vi "STATUS List (SubVI).vi"(0 "ESP Config":T1={"COM Port Input"="COM8", "Manual Command"={"Device Type"="", "Instance"="", "Command"="", "Sub-Command"="", "Parameters (Seperate by :)"=""}, "Device Type"="e", "Instance"="a", "Use Manual Command"=FALSE, "Timeout [msec]"=1000, "Read/Write Wait [msec]"=50}, 5 "Command Table Ref":refnum<vi>, 7 "STATUS Display Ref":refnum<vi>, 9 "STATUS Command Ref":refnum<vi>) -> (10 "Status Data":string, 15 "STATUS List":errorcluster)   [LabVIEW 2011]
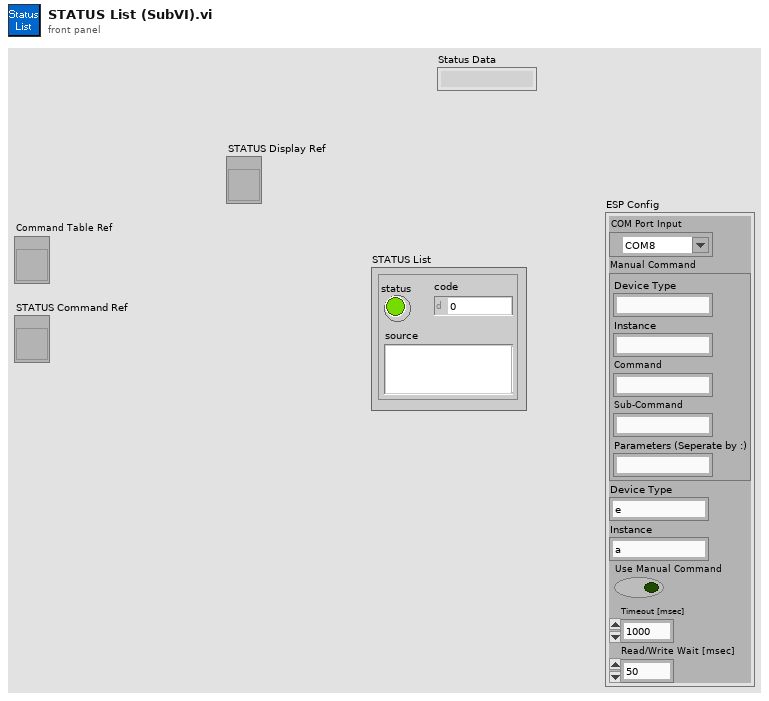
[diagram p1: front panel]
types:
  T1 = cluster{"COM Port Input":refnum<visa-resource-name>, "Manual Command":cluster{"Device Type":string, "Instance":string, "Command":string, "Sub-Command":string, "Parameters (Seperate by :)":string}, "Device Type":string, "Instance":string, "Use Manual Command":bool, "Timeout [msec]":u32, "Read/Write Wait [msec]":u32}
  T2 = cluster{"Device Type":string, "Instance":string, "Command":string, "Sub-Command":string, "Parameters (Seperate by :)":string}
  T3 = cluster{"Write Command":string, "Read String":string, "Read Bytes":u32, "Bytes at Port":u32, "Response":string, "ACK":bool, "EOT":bool, "NAK":bool, "Parameters":string[]}
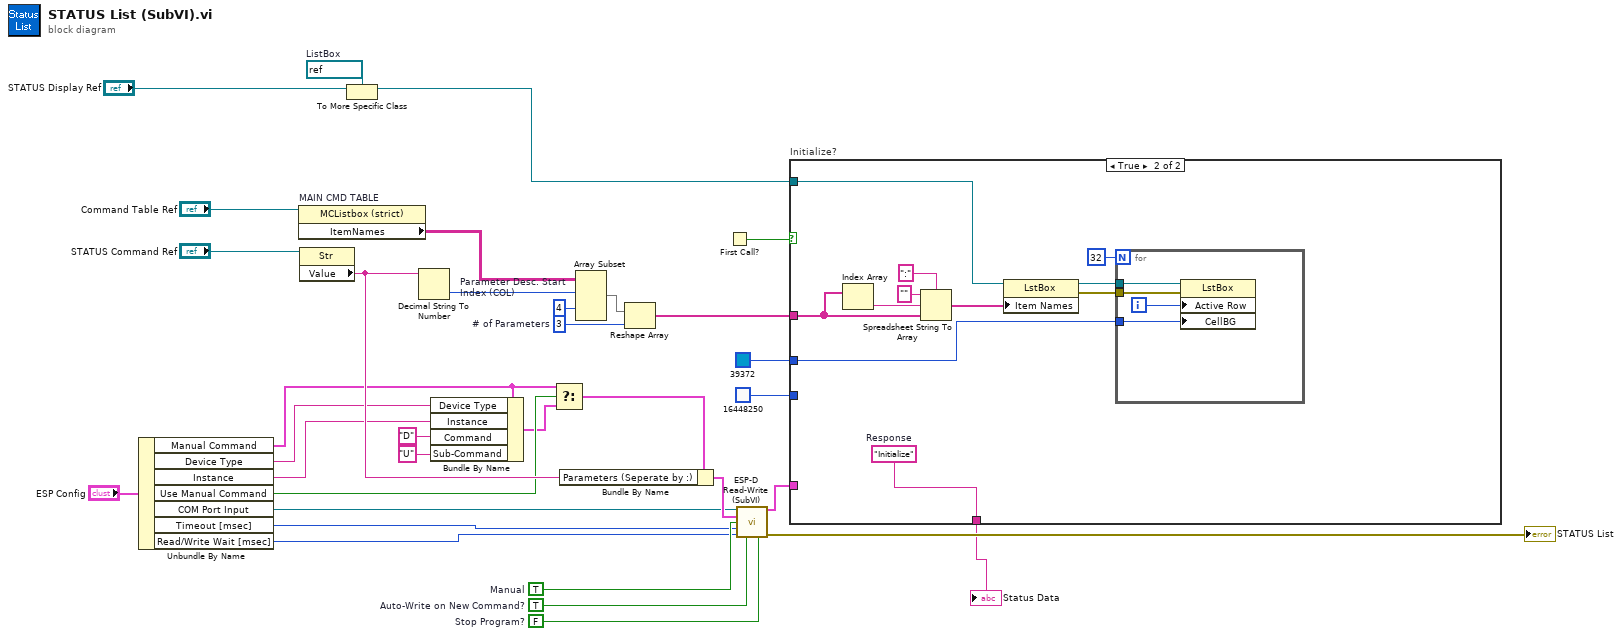
[diagram p0: block diagram]
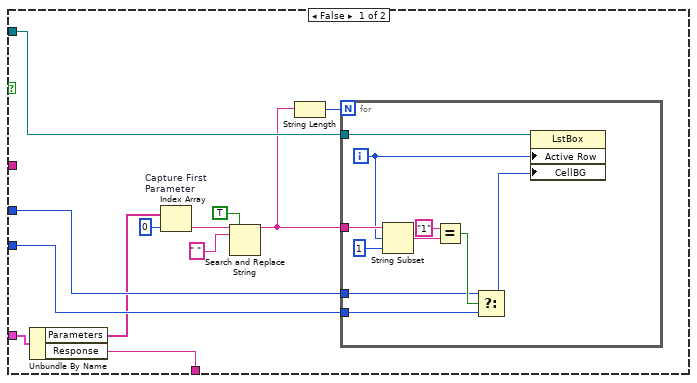
[diagram p2: hidden frame]
diagram:
  w3 = refnum<vi> refnum  # ListBox
  w26 = TRUE  # Manual
  w20 = 3  # # of Parameters
  w21 = 4  # Parameter Desc. Start Index (COL)
  w19 = FALSE  # Stop Program?
  w18 = TRUE  # Auto-Write on New Command?
  n1 = Unbundle By Name("ESP Config") -> ("Manual Command"=w7:T2, "Device Type"=w9:string, "Instance"=w8:string, "Use Manual Command"=w14:bool, "COM Port Input"=w15:refnum<visa-resource-name>, "Timeout [msec]"=w16:u32, "Read/Write Wait [msec]"=w17:u32)
  n2 = property on="MAIN CMD TABLE" class="MCListbox (strict)"(reference="Command Table Ref") -> ("ItemNames"=w5:string[][])  [unwired: 1 in, 2 out]
  n3 = property class="Str"(reference="STATUS Command Ref") -> ("Value"=w33:string)  [unwired: 1 in, 2 out]
  n4 = To More Specific Class(target class=w3, reference="STATUS Display Ref") -> (specific class reference=w1:refnum<vi>)  [unwired: 1 in, 1 out]
  n5 = Decimal String To Number(string=w33) -> (number=w25:i32)  [unwired: 2 in, 1 out]
  n6 = Bundle By Name(cluster=w7, "Device Type"=w9, "Instance"=w8, "Command"="D", "Sub-Command"="U") -> (w6:T2)
  n7 = Select(t=w7, s=w14, f=w6) -> (s? t:f=w12:T2)
  n8 = Bundle By Name(cluster=w12, "Parameters (Seperate by :)"=w33) -> (w22:T2)
  n9 = Array Subset(array=w5, index (row)=w25, index (col)=w21) -> (w23:string[][])  [unwired: 2 in]
  n10 = Reshape Array(w23, w20) -> (w27:string[])
  n11 = First Call?() -> (First Call?: T/F=w30:bool)
  n12 = call "ESP-D Read-Write (SubVI).vi"("COM Port Input"=w15, "Command Input"=w22, "Manual Write Command"=w26, "Timeout (ms)"=w16, "Write/Read Wait (ms)"=w17, "Auto-Write on New Command?"=w18, "Stop Program?"=w19) -> ("ESP Values"=w29:T3, "Error Output"=→"STATUS List":errorcluster)  [unwired: 7 in]
  n13 = case "Initialize?" shown="True" w30 {
    tunnel: w27 -> [_ w63]
    tunnel: w1 -> [w46 w67]
    tunnel: u32 39372 -> [w45 w61]
    tunnel: u32 16448250 -> [w44 _]
    tunnel: w29 -> [w43 _]
    tunnel: [w35 w57] -> w4
    frame False {
      n14 = Unbundle By Name(w43) -> ("Parameters"=w42:string[], "Response"=w35:string)
      n15 = Index Array "Capture First \nParameter"(array=w42, index=0) -> (element=w36:string)
      n16 = Search and Replace String(replace all?=TRUE ("replace all? (F)"), input string=w36, search string=" ") -> (result string=w38:string)  [unwired: 5 in, 3 out]
      n17 = String Length(string=w38) -> (length=w37:i32)
      n18 = for {
        N: w37 -> [_]
        tunnel: w38 -> [w55]
        tunnel: w46 -> [w51]
        tunnel: w45 -> [w48]
        tunnel: w44 -> [w47]
        i -> [w50]
        n19 = String Subset(string=w55, offset (0)=w50, length (rest)=1 ("length (rest)")) -> (substring=w54:string)
        n20 = Equal?(x="1", y=w54) -> (x = y?=w49:bool)
        n21 = Select(t=w48, s=w49, f=w47) -> (s? t:f=w52:u32)
        n22 = property class="LstBox"(reference=w51, "Active Row"=w50, "CellBG"=w52) -> ()  [unwired: 1 in, 2 out]
      }
    }
    frame True {
      w57 = "Initialize"  # Response
      n23 = Index Array(array=w63) -> (element=w66:string)  [unwired: 1 in]
      n24 = Spreadsheet String To Array(delimiter (Tab)=":", format string="", spreadsheet string=w66, array type (2D Dbl)=w63) -> (array=w62:string[])
      n25 = property class="LstBox"(reference=w67, "Item Names"=w62) -> (reference out=w60:refnum<vi>, error out=w59:errorcluster)  [unwired: 1 in]
      n26 = for {
        N: 32 -> [_]
        tunnel: w60 -> [w70]
        tunnel: w59 -> [w69]
        tunnel: w61 -> [w68]
        i -> [w71]
        n27 = property class="LstBox"(reference=w70, error in=w69, "Active Row"=w71, "CellBG"=w68) -> ()  [unwired: 2 out]
      }
    }
  }
  "Status Data" <- w4
